vi "Measurement_ResolveService_ServiceDescriptorContainsMeasurementInformation.vi"(8 "error in":errorcluster, 10 "expected service descriptor":T1, 11 "run service vi":refnum<vi>) -> (0 "error out":errorcluster, 2 "result":string, 3 "pass":bool)   [LabVIEW 2021, in "MeasurementServerTests.lvlib" / "Measurement Service Tests.lvlib"]
uses:
  Measurement Service Tests.lvlib
  gRPC/Generated APIs/ni/measurementlink/discovery/v1/RPC Messages/ni_measurementlink_discovery_v1_ServiceDescriptor.ctl
  gRPC/Generated APIs/ni/measurementlink/discovery/v1/RPC Messages/ni_measurementlink_discovery_v1_ServiceDescriptor_AnnotationsEntry.ctl
  Runtime/Measurements/Helpers/TypeDefs/Measurement Server User Settings.ctl
  Runtime/Measurements/Helpers/TypeDefs/Stop Server User Event.ctl
  Runtime/Measurements/Helpers/TypeDefs/Measurement Service Version.ctl
  gRPC/Generated APIs/ni/measurementlink/discovery/v1/RPC Messages/ni_measurementlink_discovery_v1_ResolveServiceRequest.ctl
  97159654-2b8c-44d4-92ef-9b7ec1865e5c.vi
  Runtime/Measurements/NI Measurement Plug-In SDK.lvlib
  Continuous Counting Client/Continuous Counting Client.lvlib
  Runtime/Clients/Discovery V1/NI Discovery V1 Client.lvlib
  gRPC/Generated APIs/ni/measurementlink/discovery/v1/ni.measurementlink.discovery.v1.api.lvlib
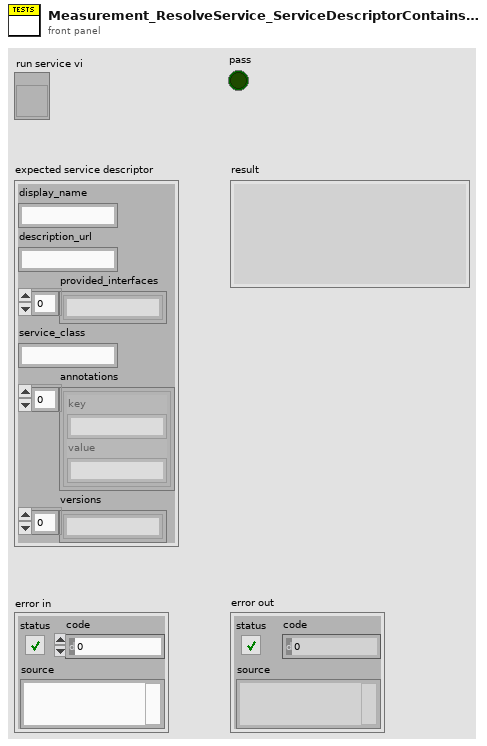
[diagram p1: front panel]
types:
  T1 = typedef "ni.measurementlink.discovery.v1.api.lvlib/ni_measurementlink_discovery_v1_ServiceDescriptor.ctl" = cluster{"display_name":string, "description_url":string, "provided_interfaces":string[], "service_class":string, "annotations":T2[], "versions":string[]}
  T2 = typedef "ni.measurementlink.discovery.v1.api.lvlib/ni_measurementlink_discovery_v1_ServiceDescriptor_AnnotationsEntry.ctl" = cluster{"key":string, "value":string}
  T3 = typedef "ni.measurementlink.discovery.v1.api.lvlib/ni_measurementlink_discovery_v1_ResolveServiceRequest.ctl" = cluster{"provided_interface":string, "service_class":string, "deployment_target":string, "version":string}
  T4 = typedef "NI Measurement Plug-In SDK.lvlib/Measurement Service Version.ctl" = enum16{"V1", "V2"}
  T5 = typedef "NI Measurement Plug-In SDK.lvlib/Measurement Server User Settings.ctl" = cluster{"stop server":T6, "measurement service versions":T4[], "show front panel":bool}
  T6 = typedef "NI Measurement Plug-In SDK.lvlib/Stop Server User Event.ctl" = refnum<user-event>
  T7 = typedef "grpc-lvsupport-release.lvlib/grpcId.ctl" = u64
  T8 = typedef "ni.measurementlink.discovery.v1.api.lvlib/ni_measurementlink_discovery_v1_ResolveServiceWithInformationResponse.ctl" = cluster{"service_location":T9, "service_descriptor":T1}
  T9 = typedef "ni.measurementlink.discovery.v1.api.lvlib/ni_measurementlink_discovery_v1_ServiceLocation.ctl" = cluster{"location":string, "insecure_port":string, "ssl_authenticated_port":string}
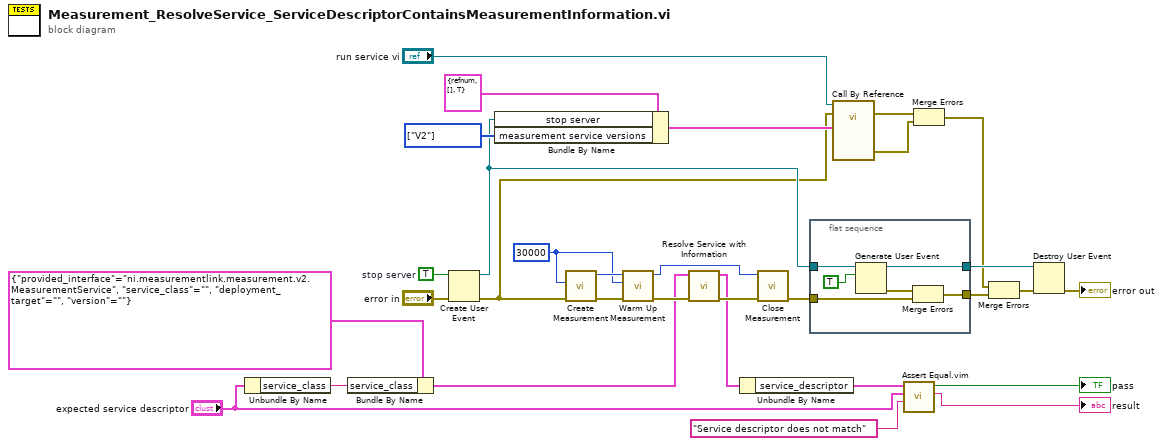
[diagram p0: block diagram]
diagram:
  w23 = 30000 ("ms timeout")
  w29 = TRUE  # stop server
  w30 = T4[] [enum."V2"] items=["V1", "V2"] ("measurement service versions")
  n1 = Unbundle By Name("expected service descriptor") -> ("service_class"=w8:string)
  n2 = Bundle By Name(cluster=T3 {"provided_interface"="ni.measurementlink.measurement.v2.MeasurementService", "service_class"="", "deployment_target"="", "version"=""} ("request data"), "service_class"=w8) -> (w4:T3)
  n3 = Create User Event(user event datatype=w29, error in="error in") -> (user event=w27:refnum<user-event>, error out=w16:errorcluster)
  n4 = Bundle By Name(cluster=T5 {"stop server"=refnum, "measurement service versions"=[], "show front panel"=TRUE} ("server settings"), "stop server"=w27, "measurement service versions"=w30) -> (w17:T5)
  n5 = call "Create Measurement.vi"("error in"=w16, "ms timeout"=w23) -> ("error out"=w25:errorcluster, "gRPCid out"=w24:T7)  [unwired: 8 in]
  n6 = call "Warm Up Measurement.vi"("error in"=w25, "timeout (ms)"=w23, "gRPC ID"=w24) -> ("error out"=w7:errorcluster, "gRPC ID out"=w12:T7)  [unwired: 6 in, 1 out]
  n7 = call "Resolve Service with Information.vi"("error in"=w7, "request data"=w4) -> ("error out"=w6:errorcluster, "response data"=w3:T8)  [unwired: 8 in]
  n8 = Unbundle By Name(w3) -> ("service_descriptor"=w2:T1)
  n9 = call "Close Measurement.vi"("error in"=w6, "gRPCid in"=w12) -> ("error out"=w26:errorcluster)  [unwired: 9 in]
  n10 = flat-sequence {
    tunnel: w27 -> [w36]
    tunnel: [w35] -> w20
    tunnel: [w34] -> w22
    tunnel: w26 -> [w33]
    frame #0 {
      n11 = Generate User Event(user event=w36, event data cluster=TRUE ("event data")) -> (user event out=w35:refnum<user-event>, error out=w37:errorcluster)  [unwired: 2 in]
      n12 = Merge Errors(w37, w33) -> (w34:errorcluster)
    }
  }
  n13 = call-by-ref "?"(reference="run service vi", error in=w16, "server settings"=w17) -> (error out=w18:errorcluster, 0:"error out"=w13:errorcluster)  [unwired: 10 in, 1 out]
  n14 = call "Assert Equal.vim"("failure message"="Service descriptor does not match", "actual value"="expected service descriptor", "expected value"=w2) -> ("message"=→"result":string, "equal?"=→"pass":bool)  [unwired: 7 in]
  n15 = Merge Errors(w18, w13) -> (w14:errorcluster)
  n16 = Merge Errors(w14, w22) -> (w21:errorcluster)
  n17 = Destroy User Event(user event=w20, error in=w21) -> (error out=→"error out":errorcluster)
